vi "Thev-Test Compute.vi"() -> ()   [LabVIEW 2015]
uses:
  Typedefs/Thev-Optimization Result.ctl
  Typedefs/Thev-Optimization Parameters.ctl
  Utility VIs/Math VIs/Linear to dB (array).vi
panel:
  in  "Probe tube":path=path "D:/Data/Calibrations/ER10XProbeA_ProbeTube.calib"
  out "Zs":cluster{"Frequency (Hz)":dbl[], "dB":dbl[]}[](graph)
  out "Result":T1
  out "Ps":cluster{"Frequency (Hz)":dbl[], "dB":dbl[]}[](graph)
  in  "folder":path=path "D:/Data/FPL/Example.2"
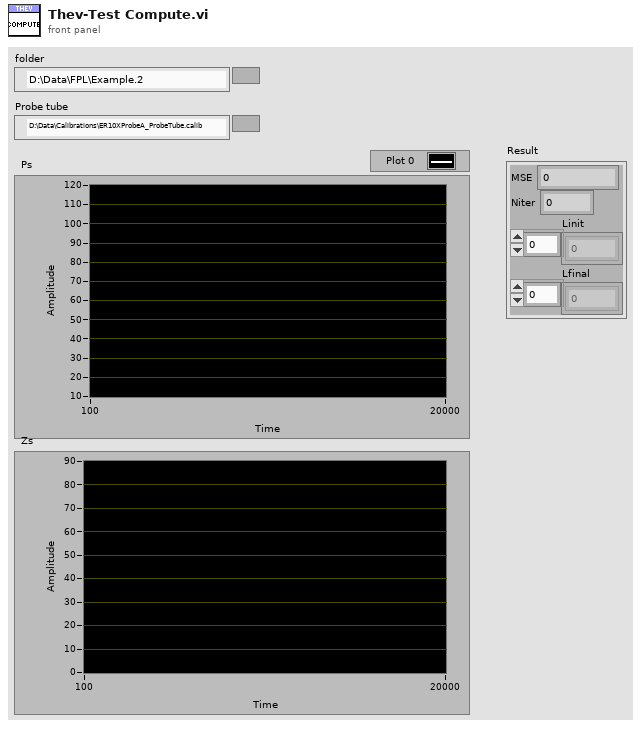
[diagram p1: front panel]
types:
  T1 = typedef "Thev-Optimization Result.ctl" = cluster{"MSE":dbl, "Niter":i32, "Linit":dbl[], "Lfinal":dbl[]}
  T2 = typedef "Thev-Optimization Parameters.ctl" = cluster{"Fmin":dbl, "Fmax":dbl}
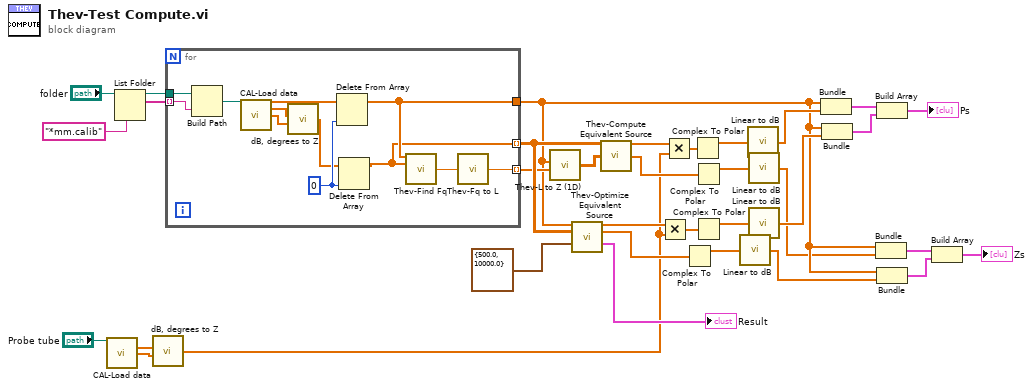
[diagram p0: block diagram]
diagram:
  n1 = call "CAL-Load data.vi"("user path"="Probe tube") -> ("Mag"=w5:dbl[], "Phase"=w4:dbl[])  [unwired: 7 in, 6 out]
  n2 = List Folder(path="folder", pattern="*mm.calib") -> (path out=w33:path, filenames=w31:string[])  [unwired: 2 in, 2 out]
  n3 = call "dB, degrees to Z.vi"("Magnitude (dB)"=w5, "Phase (degrees)"=w4) -> ("Z"=w1:cdb[])  [unwired: 5 in]
  n4 = for {
    tunnel: w33 -> [w46]
    tunnel: [w37] -> w25 mode=indexing
    tunnel: [w38] -> w14
    tunnel: w31 -> [w42] mode=indexing
    tunnel: [w39] -> w24 mode=indexing
    w36 = 0 ("index")
    n5 = Build Path(base path=w46, name or relative path=w42) -> (appended path=w45:path)
    n6 = call "CAL-Load data.vi"("user path"=w45) -> ("Frequency (Hz)"=w41:dbl[], "Mag"=w44:dbl[], "Phase"=w43:dbl[])  [unwired: 7 in, 5 out]
    n7 = call "dB, degrees to Z.vi"("Magnitude (dB)"=w44, "Phase (degrees)"=w43) -> ("Z"=w35:cdb[])  [unwired: 5 in]
    n8 = Delete From Array(array=w41, index=w36) -> (array with subset deleted=w38:dbl[])  [unwired: 1 in, 1 out]
    n9 = Delete From Array(array=w35, index=w36) -> (array with subset deleted=w37:cdb[])  [unwired: 1 in, 1 out]
    n10 = call "Thev-Find Fq.vi"("Frequency (Hz)"=w38, "Px"=w37) -> ("Fq (Hz)"=w40:dbl)  [unwired: 13 in]
    n11 = call "Thev-Fq to L.vi"("Fq (Hz)"=w40) -> ("L (mm)"=w39:dbl)
  }
  n12 = call "Thev-L to Z (1D).vi"("L (mm)"=w24, "Frequency (Hz)"=w14) -> ("Zx"=w27:cdb[][])  [unwired: 2 in]
  n13 = call "Thev-Optimize Equivalent Source.vi"("Frequency (Hz)"=w14, "Px"=w25, "Options"=T2 {"Fmin"=500.0, "Fmax"=10000.0}) -> ("Ps"=w19:cdb[], "Zs"=w12:cdb[], "Result"=→"Result":T1)  [unwired: 9 in, 1 out]
  n14 = call "Thev-Compute Equivalent Source.vi"("Px"=w25, "Zx"=w27) -> ("Ps"=w30:cdb[], "Zs"=w9:cdb[])  [unwired: 12 in]
  n15 = Multiply(x=w19, y=w1) -> (x*y=w3:cdb[])
  n16 = Multiply(x=w30, y=w1) -> (x*y=w2:cdb[])
  n17 = Complex To Polar(r * e^(i*theta)=w12) -> (r=w13:dbl[])  [unwired: 1 out]
  n18 = Complex To Polar(r * e^(i*theta)=w2) -> (r=w26:dbl[])  [unwired: 1 out]
  n19 = Complex To Polar(r * e^(i*theta)=w9) -> (r=w10:dbl[])  [unwired: 1 out]
  n20 = Complex To Polar(r * e^(i*theta)=w3) -> (r=w20:dbl[])  [unwired: 1 out]
  n21 = call-poly "Linear to dB.vi"("linear"=w13) -> ("dB"=w11:dbl[])
  n22 = call-poly "Linear to dB.vi"("linear"=w26) -> ("dB"=w29:dbl[])
  n23 = call-poly "Linear to dB.vi"("linear"=w10) -> ("dB"=w8:dbl[])
  n24 = call-poly "Linear to dB.vi"("linear"=w20) -> ("dB"=w18:dbl[])
  n25 = Bundle("Frequency (Hz)"=w14, "dB"=w29) -> (w28:cluster{"Frequency (Hz)":dbl[], "dB":dbl[]})  [unwired: 1 in]
  n26 = Bundle("Frequency (Hz)"=w14, "dB"=w18) -> (w21:cluster{"Frequency (Hz)":dbl[], "dB":dbl[]})  [unwired: 1 in]
  n27 = Bundle("Frequency (Hz)"=w14, "dB"=w8) -> (w16:cluster{"Frequency (Hz)":dbl[], "dB":dbl[]})  [unwired: 1 in]
  n28 = Build Array(w28, w21) -> (→"Ps":cluster{"Frequency (Hz)":dbl[], "dB":dbl[]}[])
  n29 = Bundle("Frequency (Hz)"=w14, "dB"=w11) -> (w15:cluster{"Frequency (Hz)":dbl[], "dB":dbl[]})  [unwired: 1 in]
  n30 = Build Array(w16, w15) -> (→"Zs":cluster{"Frequency (Hz)":dbl[], "dB":dbl[]}[])
